vi "Cluster and SubPanel Refs.vi"(7 "All Objects Refs":refnum<vi>[](array[refnum])) -> (4 "Cluster Refs":refnum<vi>[](array[refnum]), 15 "Sub Panel Refs":refnum<vi>[](array[refnum]))   [LabVIEW 2016]
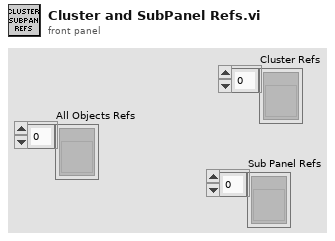
[diagram p1: front panel]
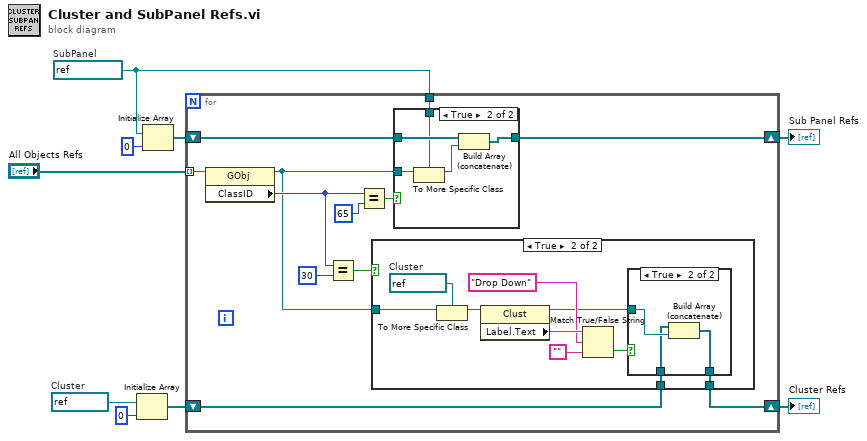
[diagram p0: block diagram]
diagram:
  w5 = refnum<vi> refnum  # Cluster
  w7 = refnum<vi> refnum  # SubPanel
  n1 = Initialize Array(w5, 0 ("dimension size")) -> (w4:refnum<vi>[])
  n2 = Initialize Array(w7, 0 ("dimension size")) -> (w8:refnum<vi>[])
  n3 = for {
    tunnel: "All Objects Refs" -> [w21] mode=indexing
    shift-right: [w17] -> w2
    shift-left: w8 -> [w18]
    tunnel: w7 -> [w16]
    shift-right: [w10] -> w3
    shift-left: w4 -> [w11]
    n4 = property class="GObj"(reference=w21) -> (reference out=w12:refnum<vi>, "ClassID"=w15:u32)  [unwired: 1 in, 1 out]
    n5 = Equal?(x=w15, y=u32 30) -> (x = y?=w13:bool)
    n6 = Equal?(x=w15, y=u32 65) -> (x = y?=w19:bool)
    n7 = case shown="True" w13 {
      tunnel: w12 -> [_ w31]
      tunnel: w11 -> [w22 w25]
      tunnel: [w22 w23] -> w10
      frame False {
      }
      frame True {
        w32 = refnum<vi> refnum  # Cluster
        n8 = To More Specific Class(target class=w32, reference=w31) -> (specific class reference=w30:refnum<vi>)  [unwired: 1 in, 1 out]
        n9 = property class="Clust"(reference=w30) -> (reference out=w24:refnum<vi>, "Label.Text"=w29:string)  [unwired: 1 in, 1 out]
        n10 = Match True/False String(2:"", 3:"Drop Down" ("true string"), 4:w29) -> (0:w26:bool)  [unwired: 1 out]
        n11 = case shown="True" w26 {
          tunnel: w25 -> [w33 w35]
          tunnel: w24 -> [_ w36]
          tunnel: [w33 w34] -> w23
          frame False {
          }
          frame True {
            n12 = Build Array (concatenate)(w35, w36) -> (w34:refnum<vi>[])
          }
        }
      }
    }
    n13 = case shown="True" w19 {
      tunnel: w18 -> [w37 w42]
      tunnel: [w37 w41] -> w17
      tunnel: w12 -> [_ w40]
      tunnel: w16 -> [_ w39]
      frame False {
      }
      frame True {
        n14 = To More Specific Class(target class=w39, reference=w40) -> (specific class reference=w38:refnum<vi>)  [unwired: 1 in, 1 out]
        n15 = Build Array (concatenate)(w42, w38) -> (w41:refnum<vi>[])
      }
    }
  }
  "Cluster Refs" <- w3
  "Sub Panel Refs" <- w2
